vi "read configuration.vi"(8 "error in (no error)":errorcluster) -> (0 "error out":errorcluster, 3 "Zone Setup Array":T1[](array[typedef]))   [LabVIEW 2015]
uses:
  Solution/Controls/Zone Setup.ctl
  Solution/Controls/Zone.ctl
  <vilib>/Utility/file.llb/Read Delimited Spreadsheet (string).vi
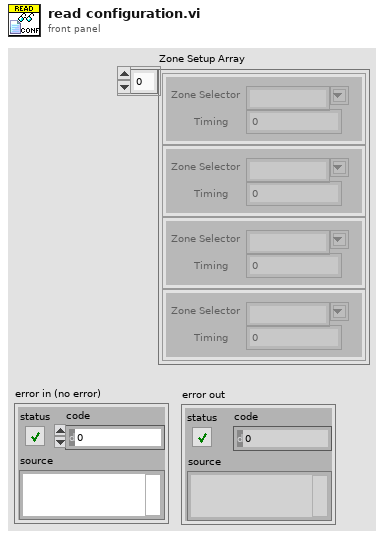
[diagram p1: front panel]
types:
  T1 = typedef "Zone Setup.ctl" = cluster{"Zone Selector":T2, "Timing":u32}
  T2 = typedef "Zone.ctl" = string
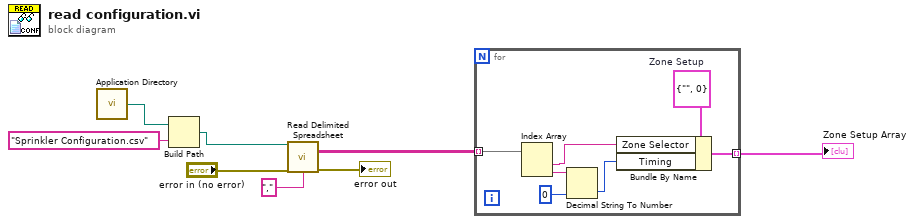
[diagram p0: block diagram]
diagram:
  n1 = call <vilib>:"Application Directory.vi"() -> ("Application Directory"=w5:path)
  n2 = Build Path(base path=w5, name or relative path="Sprinkler Configuration.csv") -> (appended path=w7:path)
  n3 = call-poly <vilib>:"Read Delimited Spreadsheet.vi"("file path (dialog if empty)"=w7, "error in (no error)"="error in (no error)", "delimiter (\\t)"="," ("delimiter (\\t)")) -> ("all rows"=w3:string[][], "error out"=→"error out":errorcluster)  [unwired: 7 in, 4 out]
  n4 = for {
    tunnel: w3 -> [w14] mode=indexing
    tunnel: [w9] -> w2 mode=indexing
    w15 = T1 {"Zone Selector"="", "Timing"=0}  # Zone Setup
    n5 = Index Array(array=w14) -> (element #1=w10:string, element #2=w13:string)  [unwired: 2 in]
    n6 = Decimal String To Number(string=w13, default (0L)=u32 0 ("Timing")) -> (number=w11:u32)  [unwired: 1 in, 1 out]
    n7 = Bundle By Name(cluster=w15, "Zone Selector"=w10, "Timing"=w11) -> (w9:T1)
  }
  "Zone Setup Array" <- w2
